vi "MotorSyncFGV.vi"(7 "Action_MotorSyncFGV":T1, 8 "error in (no error)":errorcluster, 9 "Initi MotorsToSync":enum16{"LA", "TT", "Osc"}[](array[ring])=[enum."LA", enum."TT", enum."Osc"], 11 "Motor Select":enum16{"LA", "TT", "Osc"}(ring)) -> (0 "error out":errorcluster, 1 "Status":cluster{"LA":bool, "TT":bool, "Osc":bool}, 3 "MotorSync":bool)   [LabVIEW 2017]
doc: "Developed by Kevin Thompson\nkevin@thompsonengineering.net\n\nCopyright 2018-2020\nThompson Engineering, LLC"
uses:
  DataTypes/MotorSyncFGVAction--enum.ctl
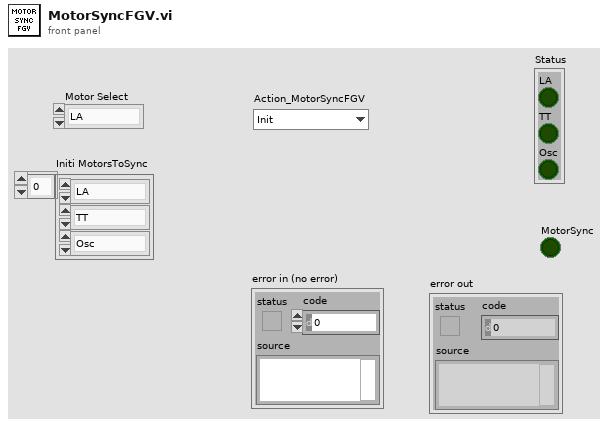
[diagram p1: front panel]
types:
  T1 = typedef "MotorSyncFGVAction--enum.ctl" = enum16{"Init", "Set", "Get"}
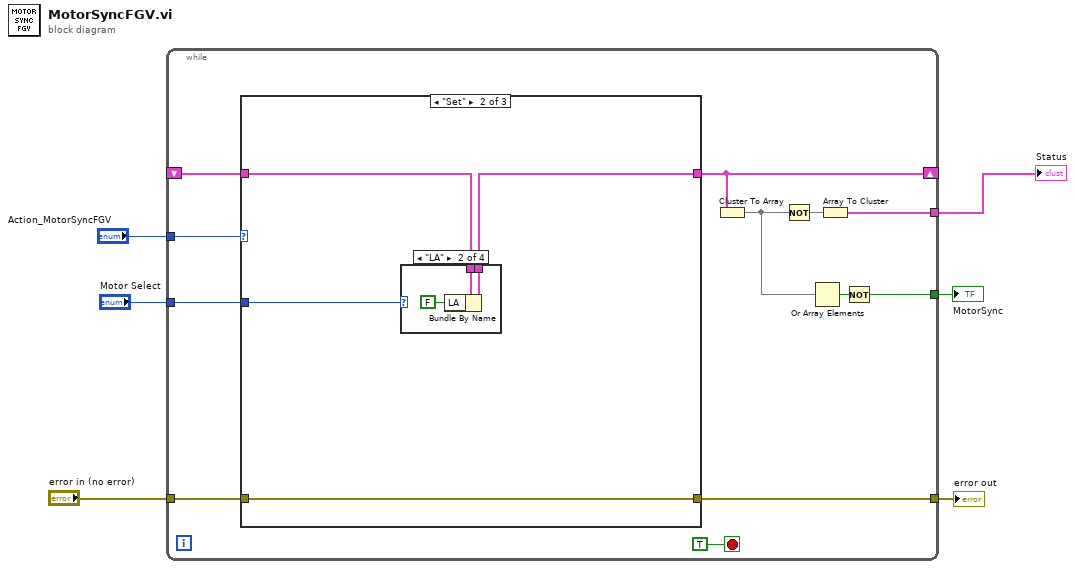
[diagram p0: block diagram]
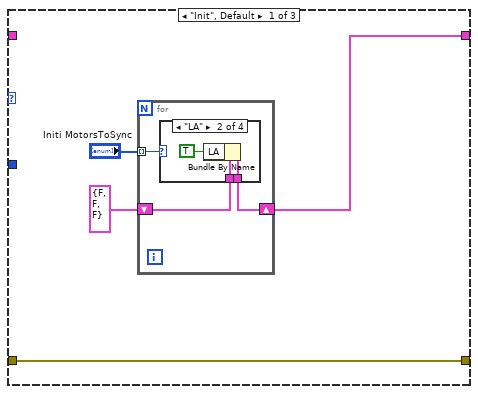
[diagram p2: hidden frame]
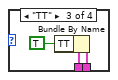
[diagram p4: hidden frame]
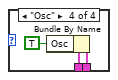
[diagram p5: hidden frame]
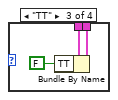
[diagram p7: hidden frame]
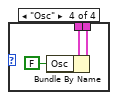
[diagram p8: hidden frame]
diagram:
  n1 = while {
    tunnel: "Action_MotorSyncFGV" -> [w17]
    tunnel: [w10] -> w5
    tunnel: "error in (no error)" -> [w15]
    tunnel: [w14] -> w3
    shift-right: [w12] -> _
    shift-left: _ -> [w13]
    tunnel: "Motor Select" -> [w11]
    tunnel: [w7] -> w1
    stop <- TRUE stop-if-true
    n2 = case shown="\"Set\"" w17 {
      tunnel: w15 -> [w22 w39 w51]
      tunnel: [w22 w39 w51] -> w14
      tunnel: [w19 w37 w50] -> w12
      tunnel: w13 -> [_ w38 w50]
      tunnel: w11 -> [_ w36 _]
      frame "Init", Default {
        n3 = for {
          tunnel: "Initi MotorsToSync" -> [w24] mode=indexing
          shift-right: [w23] -> w19
          shift-left: cluster{"LA":bool, "TT":bool, "Osc":bool} {"LA"=FALSE, "TT"=FALSE, "Osc"=FALSE} ("MotorsToSync") -> [w25]
          n4 = case shown="\"LA\"" w24 {
            tunnel: w25 -> [w26 w29 w32 w35]
            tunnel: [w26 w27 w30 w33] -> w23
            frame Default {
            }
            frame "LA" {
              n5 = Bundle By Name(cluster=w29, "LA"=TRUE) -> (w27:cluster{"LA":bool, "TT":bool, "Osc":bool})
            }
            frame "TT" {
              n6 = Bundle By Name(cluster=w32, "TT"=TRUE) -> (w30:cluster{"LA":bool, "TT":bool, "Osc":bool})
            }
            frame "Osc" {
              n7 = Bundle By Name(cluster=w35, "Osc"=TRUE ("TT")) -> (w33:cluster{"LA":bool, "TT":bool, "Osc":bool})
            }
          }
        }
      }
      frame "Set" {
        n8 = case shown="\"LA\"" w36 {
          tunnel: w38 -> [w40 w42 w45 w48]
          tunnel: [w40 w41 w44 w47] -> w37
          frame Default {
          }
          frame "LA" {
            n9 = Bundle By Name(cluster=w42, "LA"=FALSE) -> (w41:cluster{"LA":bool, "TT":bool, "Osc":bool})
          }
          frame "TT" {
            n10 = Bundle By Name(cluster=w45, "TT"=FALSE) -> (w44:cluster{"LA":bool, "TT":bool, "Osc":bool})
          }
          frame "Osc" {
            n11 = Bundle By Name(cluster=w48, "Osc"=FALSE ("TT")) -> (w47:cluster{"LA":bool, "TT":bool, "Osc":bool})
          }
        }
      }
      frame "Get" {
      }
    }
    n12 = Cluster To Array(cluster=w12) -> (array=w9:bool[])
    n13 = Not(x=w9) -> (.not. x?=w8:bool[])
    n14 = Or Array Elements(Boolean array=w9) -> (logical OR=w16:bool)
    n15 = Array To Cluster(array=w8) -> (cluster=w7:cluster{"[0]":bool, "[1]":bool, "[2]":bool})
    n16 = Not(x=w16) -> (.not. x?=w10:bool)
  }
  "MotorSync" <- w5
  "error out" <- w3
  "Status" <- w1
